vi "Load_Traverse_file.vi"(0 "Setup filename":path) -> (3 "Setup filename Out":path, 4 "Jump Bad Positions":bool, 5 "Table":T2[](array[typedef]) {"Row Duration (mins)" format="%#.1f"; "Row No" min=0; "Trace Gas Concentration (%)" min=0.0 format="%#.2f"; "Emission Rate (l/min)" format="%#.2f"; "Tunnel Speed" format="%#.2f"; "Start X" format="%#.2f"; "Start Y" format="%#.2f"; "Start Z" format="%#.2f"; "End X" format="%#.2f"; "End Y" format="%#.2f"; "End Z" format="%#.2f"; "Averaging time (min)" min=0.0 format="%#.2f"}, 6 "Work in Tunnel Coordinates?":T1)   [LabVIEW 2012]
uses:
  Traverse_cluster.ctl
  Spacing.ctl
  Controls/Multi_run_mode.ctl
  Controls/Tunnel_Coordinates.ctl
panel:
  # "HD:Users"
  # "HD:Users"
  # "X           Y            Z"
  # "Start"
  # "End"
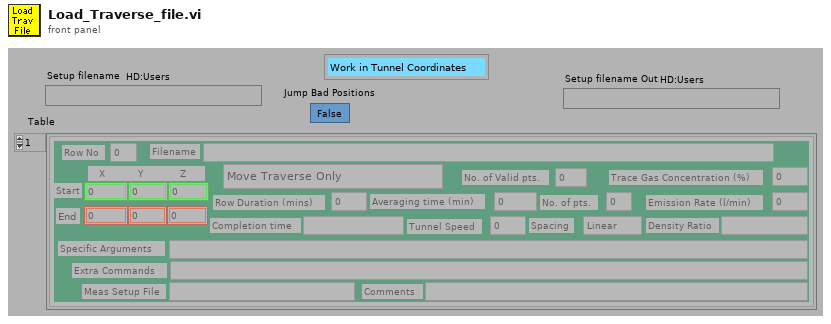
[diagram p1: front panel]
types:
  T1 = typedef "Tunnel_Coordinates.ctl" = enum16{"Work in Tunnel Coordinates", "Work in Model Coordinates"}
  T2 = typedef "Traverse_cluster.ctl" = cluster{"Start X":dbl, "Start Y":dbl, "Start Z":dbl, "End X":dbl, "End Y":dbl, "End Z":dbl, "No. of pts.":i32, "Spacing":T3, "Filename":path, "Tunnel Speed":dbl, "Averaging time (min)":dbl, "Extra Commands":string, "Specific Arguments":string, "Emission Rate (l/min)":dbl, "Trace Gas Concentration (%)":dbl, "Density Ratio":string, "Comments":string, "Row No":i32, "Row Type Selector":T4, "Completion time":string, "Row Duration (mins)":dbl, "No. of Valid pts.":i32, "Meas Setup File":string}
  T3 = typedef "Spacing.ctl" = enum16{"Linear", "Log", "Gauss", "Specified", "N/A"}
  T4 = typedef "Multi_run_mode.ctl" = enum16{"Move Traverse Only", "Set Tunnel Speed Only", "Set Source Only", "Set Measurement Conditions", "Single Measurement", "Vertical Profile", "Lateral Profile", "Longitudinal Profile", "Explore Volume", "Multi-Axis Profile", "Auto Calibrate", "Meas Fast FID Bkgnd", "Check Beam Power", "Scanning Valve Measurement", "Run VI Named:", "Set ADAM Ch", "Wait (minutes)", "Send Message", "Synchronize With:", "Fall Back to this Row", "Turn Off Row Repeating", "Blank Row", "Traverse 3D Volume"}
  T5 = enum16{"All Channel Names", "Valid Channel Names"}
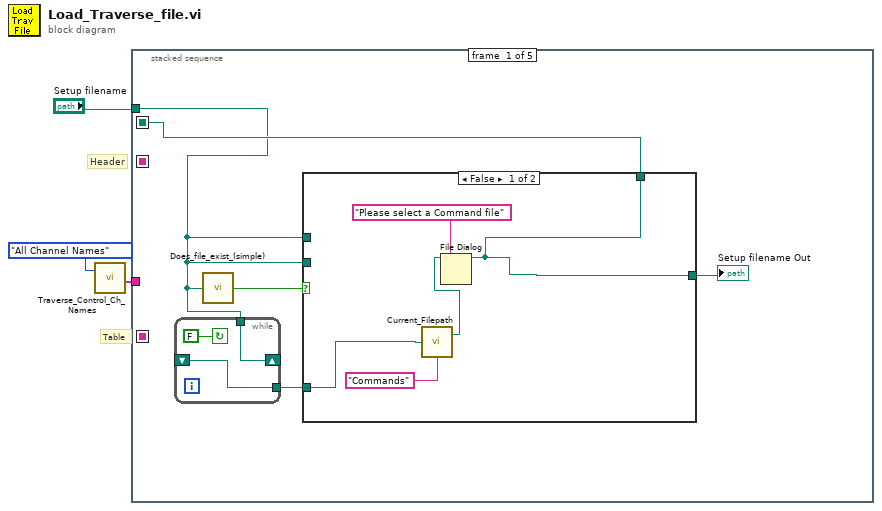
[diagram p0: block diagram]
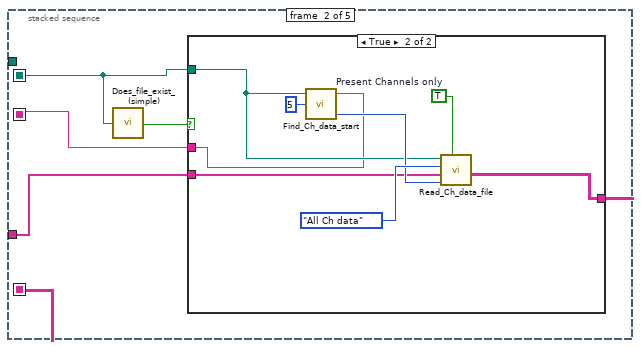
[diagram p3: hidden frame]
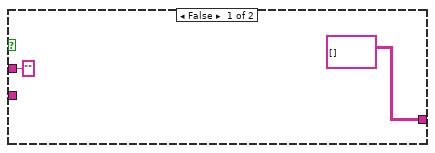
[diagram p4: hidden frame]
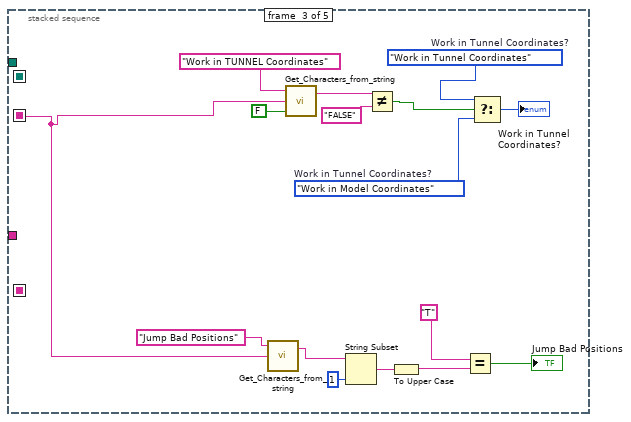
[diagram p5: hidden frame]
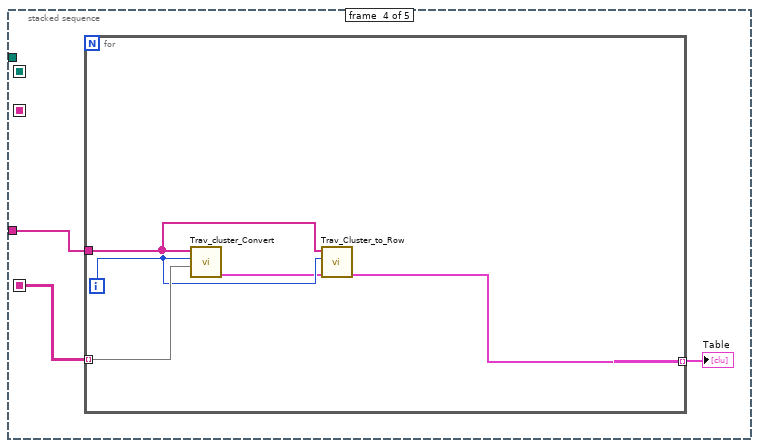
[diagram p6: hidden frame]
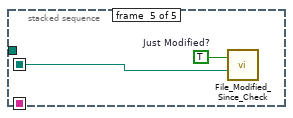
[diagram p7: hidden frame]
diagram:
  # "Header"
  # "Table"
  n1 = call "Traverse_Control_Ch_Names.vi"("Mode"=T5."All Channel Names") -> ("Channel names"=w2:string[])  [unwired: 1 in]
  n2 = stacked-sequence {
    seq-local: [_ w23 _ _ _] -> [_ _ _ w52 _]
    seq-local: [_ w22 _ _ _] -> [_ _ w40 _ _]
    seq-local: [w8 _ _ _ _] -> [_ w20 _ _ w58]
    tunnel: "Setup filename" -> [w4 _ _ _ _]
    tunnel: w2 -> [_ w19 _ w51 _]
    frame #0 {
      n3 = while {
        tunnel: [w10] -> w5
        tunnel: w4 -> [w11]
        shift-left: _ -> [w10]
        shift-right: [w11] -> _
        stop <- FALSE continue-if-true
      }
      n4 = call "Does_file_exist_(simple).vi"("Pathname"=w4) -> ("exists?"=w6:bool)
      n5 = case shown="False" w6 {
        tunnel: w4 -> [_ w18]
        tunnel: [w15 w18] -> w8
        tunnel: [w15 w17] -> w7
        tunnel: w4 -> [_ w17]
        tunnel: w5 -> [w13 _]
        frame False {
          n6 = call "Current_Filepath.vi"("Filename in"=w13, "Data Type"="Commands") -> ("Directory"=w12:path)  [unwired: 1 out]
          n7 = File Dialog(7:"Please select a Command file" ("prompt"), 11:w12) -> (3:w15:path)  [unwired: 1 in, 7 out]
        }
        frame True {
        }
      }
      "Setup filename Out" <- w7
    }
    frame #1 {
      n8 = call "Does_file_exist_(simple).vi"("Pathname"=w20) -> ("exists?"=w21:bool)
      n9 = case shown="True" w21 {
        tunnel: [string[][] [] w28] -> w23
        tunnel: ["" ("character string") w29] -> w22
        tunnel: w20 -> [_ w30]
        tunnel: w19 -> [_ w27]
        frame False {
        }
        frame True {
          w33 = TRUE  # Present Channels only
          n10 = call "Find_Ch_data_start.vi"("Approx No Of Columns"=5, "Filename"=w30) -> ("Start of read offset output"=w31:i32, "String before data"=w29:string)  [unwired: 1 in, 1 out]
          n11 = call "Read_Ch_data_file.vi"("Present Channels only"=w33, "Start of read offset (chars.: 0)"=w31, "Present Channels"=w27, "Output"=enum16{"All Ch data", "The last few rows"}."All Ch data", "Filename"=w30) -> ("Channel Values"=w28:string[][])  [unwired: 4 out]
        }
      }
    }
    frame #2 {
      w43 = Tunnel_Coordinates."Work in Model Coordinates"  # Work in Tunnel Coordinates?
      w45 = Tunnel_Coordinates."Work in Tunnel Coordinates"  # Work in Tunnel Coordinates?
      n12 = call "Get_Characters_from_string.vi"("Input string"=w40, "Variable name"="Jump Bad Positions" ("Label for characters")) -> ("Value"=w35:string)  [unwired: 1 in, 1 out]
      n13 = call "Get_Characters_from_string.vi"("Show Dialog?"=FALSE, "Input string"=w40, "Variable name"="Work in TUNNEL Coordinates" ("Label for characters")) -> ("Value"=w48:string)  [unwired: 1 out]
      n14 = String Subset(string=w35, length (rest)=1 ("length")) -> (substring=w37:string)  [unwired: 1 out]
      n15 = Not Equal?(x=w48, y="FALSE") -> (x != y?=w46:bool)
      n16 = To Upper Case(1:w37) -> (0:w36:string)
      n17 = Equal?(x="T", y=w36) -> (x = y?=→"Jump Bad Positions":bool)
      n18 = Select(t=w45, s=w46, f=w43) -> (s? t:f=→"Work in Tunnel Coordinates?":T1)
    }
    frame #3 {
      n19 = for {
        tunnel: w52 -> [w57] mode=indexing
        tunnel: [w54] -> w50 mode=indexing
        tunnel: w51 -> [w56]
        i -> [w55]
        n20 = call "Trav_cluster_Convert.vi"("Channel Values In"=w57, "Row Number"=w55, "Channel names"=w56) -> ("Traverse line Out"=w53:T2)  [unwired: 1 in, 3 out]
        n21 = call "Trav_Cluster_to_Row.vi"("Traverse line in"=w53, "Row Number"=w55, "Channel names"=w56) -> ("Traverse line Out"=w54:T2)  [unwired: 4 out]
      }
      "Table" <- w50
    }
    frame #4 {
      w59 = TRUE  # Just Modified?
      n22 = call "File_Modified_Since_Check.vi"("Pathname"=w58, "Just Modified?"=w59) -> ()  [unwired: 1 out]
    }
  }
